vi "Init_config.vi"(7 "error in":errorcluster) -> (4 "Hexapod initialized?":bool, 6 "Identification":string, 8 "Conn. Axes":string[](array[string]), 10 "Position":dbl[](array[numeric]) format="%.6f", 15 "error out":errorcluster)   [LabVIEW 2011]
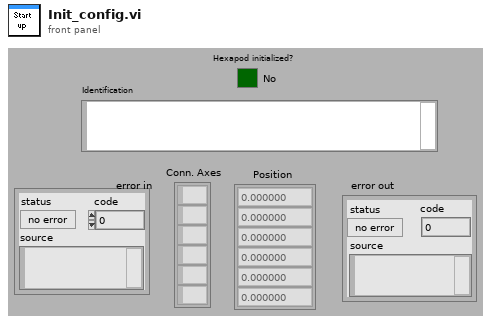
[diagram p1: front panel]
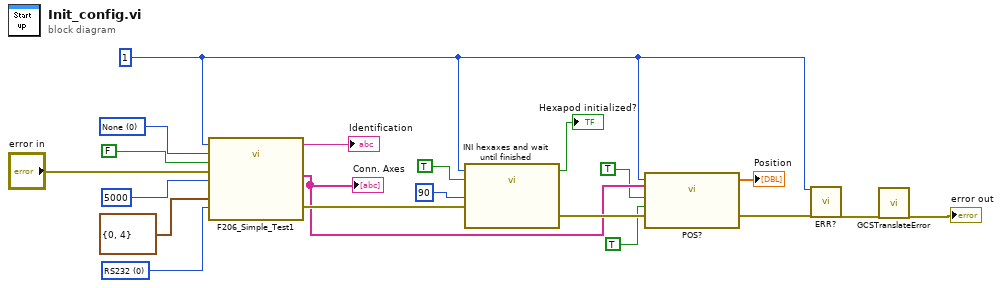
[diagram p0: block diagram]
diagram:
  w16 = u16 0 items=["RS232", "GPIB"] ("Interface")
  w20 = u16 0 items=["None", "One axis (A)", "Two axes (A and B)"] ("How many additional axes?")
  w4 = 1 ("System no.")
  n1 = call "F206_Simple_Test1.vi"("System no."=w4, "How many additional axes?"=w20, "Is a NanoCube present?"=FALSE, "error in"="error in", "Interface"=w16, "Timeout"=u32 5000, "RS232 settings"=cluster{"Portnumber":u16, "Baudrate":u16} {"Portnumber"=0, "Baudrate"=4}) -> ("Identification"=→"Identification":string, "Conn. Axes"=w9:string[], "error out"=w14:errorcluster)  [unwired: 10 in]
  "Conn. Axes" <- w9
  n2 = call "INI hexaxes and wait until finished.vi"("System no."=w4, "INI hexapod?"=TRUE, "Timeout, sec"=u32 90, "error in"=w14) -> ("Hexapod initialized?"=→"Hexapod initialized?":bool, "error out"=w10:errorcluster)  [unwired: 12 in, 2 out]
  n3 = call "POS?.vi"("System no."=w4, "Axes to query"=w9, "All axes?"=TRUE, "Axis identifier?"=TRUE, "error in"=w10) -> ("Position"=→"Position":dbl[], "error out"=w5:errorcluster)  [unwired: 13 in]
  n4 = call "ERR?.vi"("System no."=w4, "error in"=w5) -> ("error out"=w3:errorcluster)  [unwired: 16 in, 1 out]
  n5 = call "GCSTranslateError.vi"("error in"=w3) -> ("error out"=→"error out":errorcluster)  [unwired: 16 in, 2 out]
